vi "From Input Task.vi"   [LabVIEW 2022 SP3, in "DAAG task conversion.lvlib"]
uses:
  DAAG task conversion.lvlib
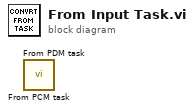
[diagram p0: block diagram]
diagram:
  n1 = call "From PCM task.vi"() -> ()  [unwired: 11 in, 1 out]
  n2 = call "From PDM task.vi"() -> ()  [unwired: 11 in, 1 out]
